vi "Constant getFolderPath.vi"(2 "error in (no error)":errorcluster, 3 "folder name":T1=enum."system_log") -> (0 "error out":errorcluster, 1 "folder path":path)   [LabVIEW 2018]
uses:
  AccessFolderName.ctl
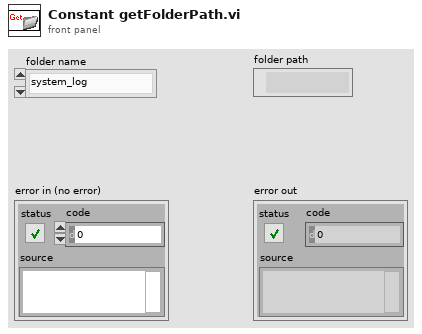
[diagram p1: front panel]
types:
  T1 = typedef "AccessFolderName.ctl" = enum16{"None", "system_log", "ui_log", "msdata", "method", "d999_param"}
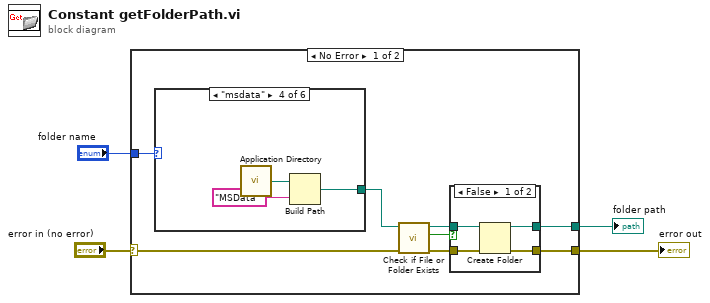
[diagram p0: block diagram]
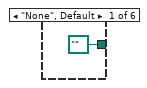
[diagram p3: hidden frame]
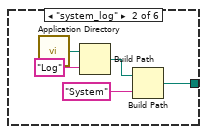
[diagram p4: hidden frame]
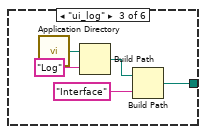
[diagram p5: hidden frame]
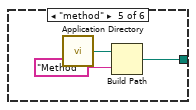
[diagram p6: hidden frame]
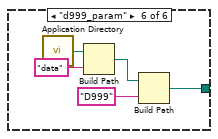
[diagram p7: hidden frame]
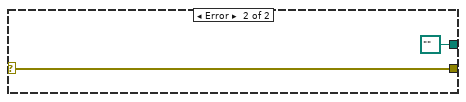
[diagram p8: hidden frame]
diagram:
  n1 = case shown="No Error" "error in (no error)" {
    selector: "error in (no error)" -> [w8 w41]
    tunnel: "folder name" -> [w12 _]
    tunnel: [w5 w41] -> w2
    tunnel: [w6 path "" ("dup path")] -> w1
    frame No Error {
      n2 = case shown="\"msdata\"" w12 {
        tunnel: [path "" ("appended path") w20 w25 w30 w33 w38] -> w7
        frame "None", Default {
        }
        frame "system_log" {
          n3 = call <vilib>:"Application Directory.vi"() -> ("Application Directory"=w23:path)
          n4 = Build Path(base path=w23, name or relative path="Log") -> (appended path=w22:path)
          n5 = Build Path(base path=w22, name or relative path="System") -> (appended path=w20:path)
        }
        frame "ui_log" {
          n6 = call <vilib>:"Application Directory.vi"() -> ("Application Directory"=w28:path)
          n7 = Build Path(base path=w28, name or relative path="Log") -> (appended path=w27:path)
          n8 = Build Path(base path=w27, name or relative path="Interface") -> (appended path=w25:path)
        }
        frame "msdata" {
          n9 = call <vilib>:"Application Directory.vi"() -> ("Application Directory"=w31:path)
          n10 = Build Path(base path=w31, name or relative path="MSData") -> (appended path=w30:path)
        }
        frame "method" {
          n11 = call <vilib>:"Application Directory.vi"() -> ("Application Directory"=w34:path)
          n12 = Build Path(base path=w34, name or relative path="Method") -> (appended path=w33:path)
        }
        frame "d999_param" {
          n13 = call <vilib>:"Application Directory.vi"() -> ("Application Directory"=w39:path)
          n14 = Build Path(base path=w39, name or relative path="data") -> (appended path=w37:path)
          n15 = Build Path(base path=w37, name or relative path="D999") -> (appended path=w38:path)
        }
      }
      n16 = call <vilib>:"Check if File or Folder Exists.vi"("error in (no error)"=w8, "path"=w7) -> ("error out"=w9:errorcluster, "file or folder exists?"=w11:bool, "dup path"=w10:path)  [unwired: 7 in]
      n17 = case shown="False" w11 {
        tunnel: w10 -> [w16 w18]
        tunnel: w9 -> [w15 w17]
        tunnel: [w14 w18] -> w6
        tunnel: [w13 w17] -> w5
        frame False {
          n18 = Create Folder(path (use dialog)=w16, error in=w15) -> (created path=w14:path, error out=w13:errorcluster)  [unwired: 1 in, 1 out]
        }
        frame True {
        }
      }
    }
    frame Error {
    }
  }
  "error out" <- w2
  "folder path" <- w1
